vi "exmpl_File_Upload_Helper.vi"(8 "error in":errorcluster caption="error out") -> (0 "error out":errorcluster, 2 "output cluster":T1)   [LabVIEW 2013, in "daqio minimal.lvlib"]
uses:
  daqio minimal.lvlib
panel:
  out "selected path":path
  in  "Confirm File Upload":bool
  in  "File Type":string(combo)="binary"
  in  "File Label (File Name by default)":string
  # "Please select a file to upload in the \nfile dialog and select its type here. \nIf you are not sure which type to\nselect, choose \"binary\"."
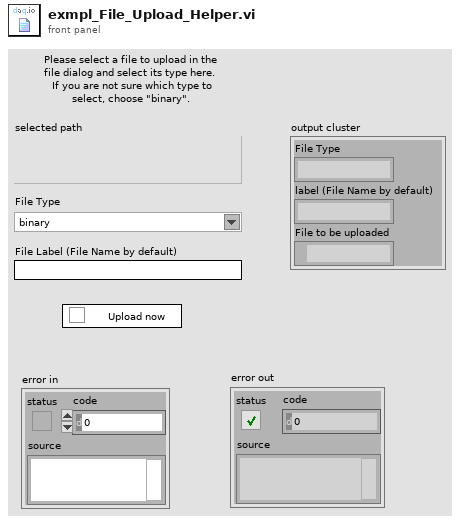
[diagram p1: front panel]
types:
  T1 = cluster{"File Type":string, "label (File Name by default)":string, "File to be uploaded":path}
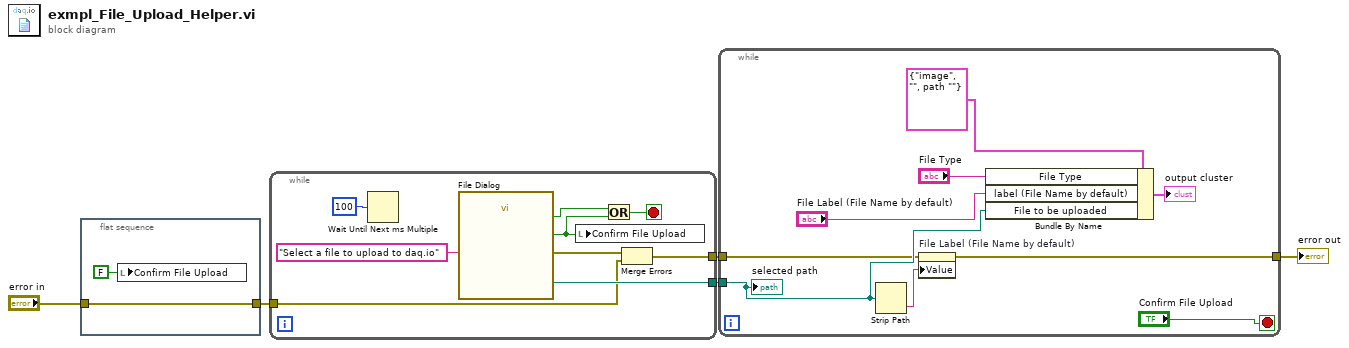
[diagram p0: block diagram]
diagram:
  n1 = flat-sequence {
    tunnel: "error in" -> [w6]
    tunnel: [w6] -> w1
    frame #0 {
      n2 = local write "Confirm File Upload"(FALSE ("Confirm File Upload")) -> ()
    }
  }
  n3 = while {
    tunnel: [w16] -> w4
    tunnel: [w11] -> w3
    tunnel: w1 -> [w10]
    stop <- w9 stop-if-true
    n4 = Wait Until Next ms Multiple(millisecond multiple=u32 100) -> ()  [unwired: 1 out]
    n5 = call "File Dialog"("prompt"="Select a file to upload to daq.io") -> ("selected path"=w16:path, "exists"=w14:bool, "cancelled"=w8:bool, "error out"=w15:errorcluster)  [unwired: 11 in]
    n6 = local write "Confirm File Upload"(w8) -> ()
    n7 = Or(x=w14, y=w8) -> (x .or. y?=w9:bool)
    n8 = Merge Errors(w15, w10) -> (w11:errorcluster)
  }
  n9 = while {
    tunnel: [w25] -> w5
    tunnel: w4 -> [w20]
    tunnel: w3 -> [w18]
    stop <- "Confirm File Upload" stop-if-true
    n10 = Strip Path(path=w20) -> (name=w19:string)  [unwired: 1 out]
    n11 = property on="File Label (File Name by default)" class="Str"(error in=w18, "Value"=w19) -> (error out=w25:errorcluster)  [unwired: 1 in, 1 out]
    n12 = Bundle By Name(cluster=T1 {"File Type"="image", "label (File Name by default)"="", "File to be uploaded"=path ""} ("File to upload"), "File Type"="File Type", "label (File Name by default)"="File Label (File Name by default)", "File to be uploaded"=w20) -> (→"output cluster":T1)
    "selected path" <- w20
  }
  "error out" <- w5
